vi "PPS User Interface.vi"() -> ()   [LabVIEW 2023, in "GUI.lvlib" / "Diagnostic.lvlib"]
uses:
  Diagnostic.lvlib
  HardwareAbstractionLayer_LVOOP/Database/SQL Public VI/Control/DB Options.ctl
  Control/PPS Configure UI.ctl
  HardwareAbstractionLayer_LVOOP/PowerSupply/Control/PPS Configure Data.ctl
  HardwareAbstractionLayer_LVOOP/PowerSupply/PowerSupply.lvclass
  HardwareAbstractionLayer_LVOOP/Database/Database.lvclass
panel:
  in  "Stop":bool caption="Blank"
  in  "Apply":bool caption="Blank"
  in  "PPS Driver":T1(ring)
  out "error out":errorcluster
  in  "error in":errorcluster
  in  "PPS Operation":T2(tab)
  in  "PowerSupply Instrument":T3(ring)
  out "Status":bool
  out "Self-Test Result Message":string
  in  "OCP Delays (S)":dbl=1.0 caption="Absolute Resolution (1E-6)" format="%.2p"
  in  "OVP Delays (S)":dbl=1.0 caption="Absolute Resolution (1E-6)" format="%.2p"
  in  "Current Limit OCP (A)":dbl=8.0 caption="Absolute Resolution (1E-6)" format="%.2p"
  in  "Voltage Limit  (V)":dbl=15.0 caption="Absolute Resolution (1E-6)" format="%.2p"
  in  "Current  Limit  (A)":dbl=6.0 caption="Absolute Resolution (1E-6)" format="%.2p"
  in  "Voltage Limit OVP (V)":dbl=15.0 caption="Absolute Resolution (1E-6)" format="%.2p"
  in  "Current Level (A)":dbl=8.0 caption="Absolute Resolution (1E-6)" format="%.2p"
  in  "Voltage Level (V)":dbl=12.0 format="%#.2g"
  in  "Output Priority Mode":u16(ring) items=["Voltage", "Current"]
  in  "Output":bool
  in  "OVP":bool
  in  "OCP":bool
  out "Current (A)":dbl format="%_4f"
  out "Voltage (V)":dbl format="%_4f"
  # "Programmbale Power Supply"
  # "Operation:"
  # "Self Test is Enabled by selecting this opeartion"
  # "PPS Close Operation will be executing \n        by selecting this opeartion"
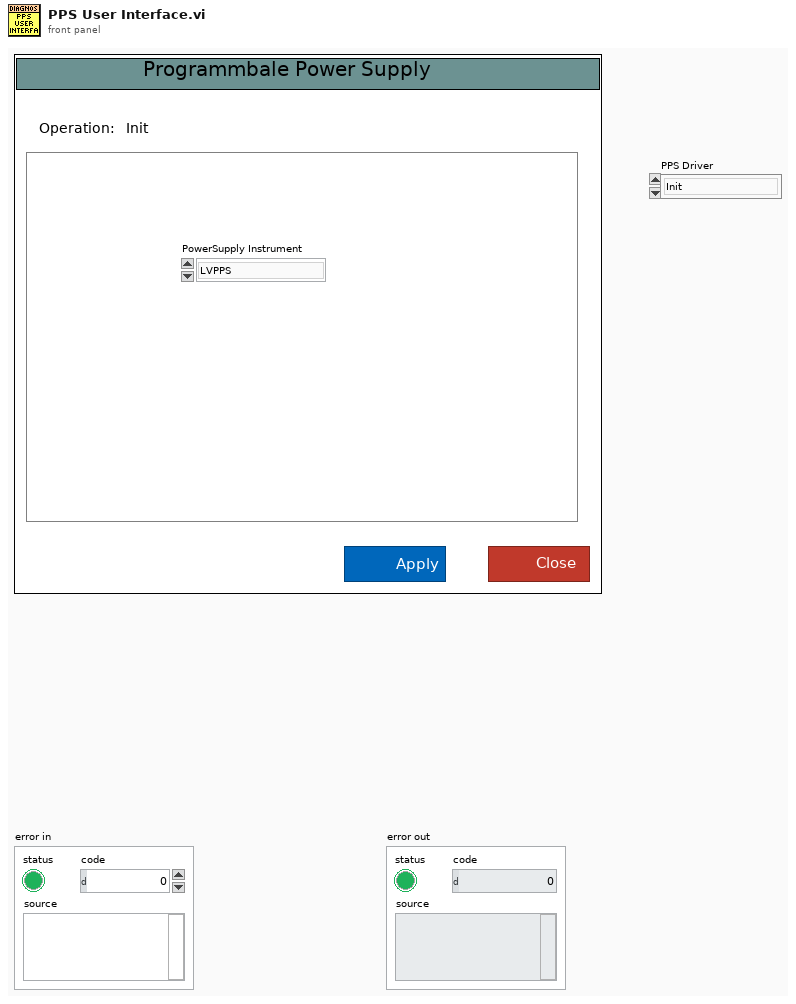
[diagram p1: front panel]
types:
  T1 = enum32{"Init", "Self Test", "Configure", "Measure", "Close"}
  T2 = enum32{"Init", "Self Test", "Configure", "Measure Current", "Measure Voltage", "Close"}
  T3 = enum16{"LVPPS", "HVPPS1", "HVPPS2", "HVPPS3", "HVPPS4", "HVPPS5", "HVPPS6"}
  T4 = typedef "HardwareAbstractionLayer_LVOOP.lvlib/Database.lvclass/DB Options.ctl" = enum16{"Init", "Select Data", "Insert Data", "Update Data", "Delete Data", "Execute Query", "Create Schema", "Create Table", "List Tables", "List Columns", "Close"}
  T5 = typedef "GUI.lvlib/Diagnostic.lvlib/PPS Configure UI.ctl" = cluster{"PPS Operation":enum32{"Init", "Self Test", "Configure", "Measure", "Close"}, "PowerSupply Instrument":enum16{"LVPPS", "HVPPS1", "HVPPS2", "HVPPS3", "HVPPS4", "HVPPS5", "HVPPS6"}, "Configure":T6}
  T6 = typedef "HardwareAbstractionLayer_LVOOP.lvlib/PowerSupply.lvclass/PPS Configure Data.ctl" = cluster{"Voltage Level (0.0 V)":dbl, "CURRent Limit (0.0 A)":dbl, "OVP LEVEL (0V)":dbl, "OCP LEVEL (0A)":dbl, "Enable OVP (T: Enable)":bool, "Enable OCP (T: Enable)":bool, "Enable Output ":bool, "Delays OCP":dbl, "Delays OVP":dbl, "Mode(0:Voltage)":u16, "CURRent Level (0.0 A)":dbl, "Voltage Limit (0.0 V)":dbl}
  T7 = typedef "GUI.lvlib/Diagnostic.lvlib/PPS Out Data UI.ctl" = cluster{"Self-Test Result Message":string, "Actual Voltage Level (V)":dbl, "Actual Current Limit (A)":dbl}
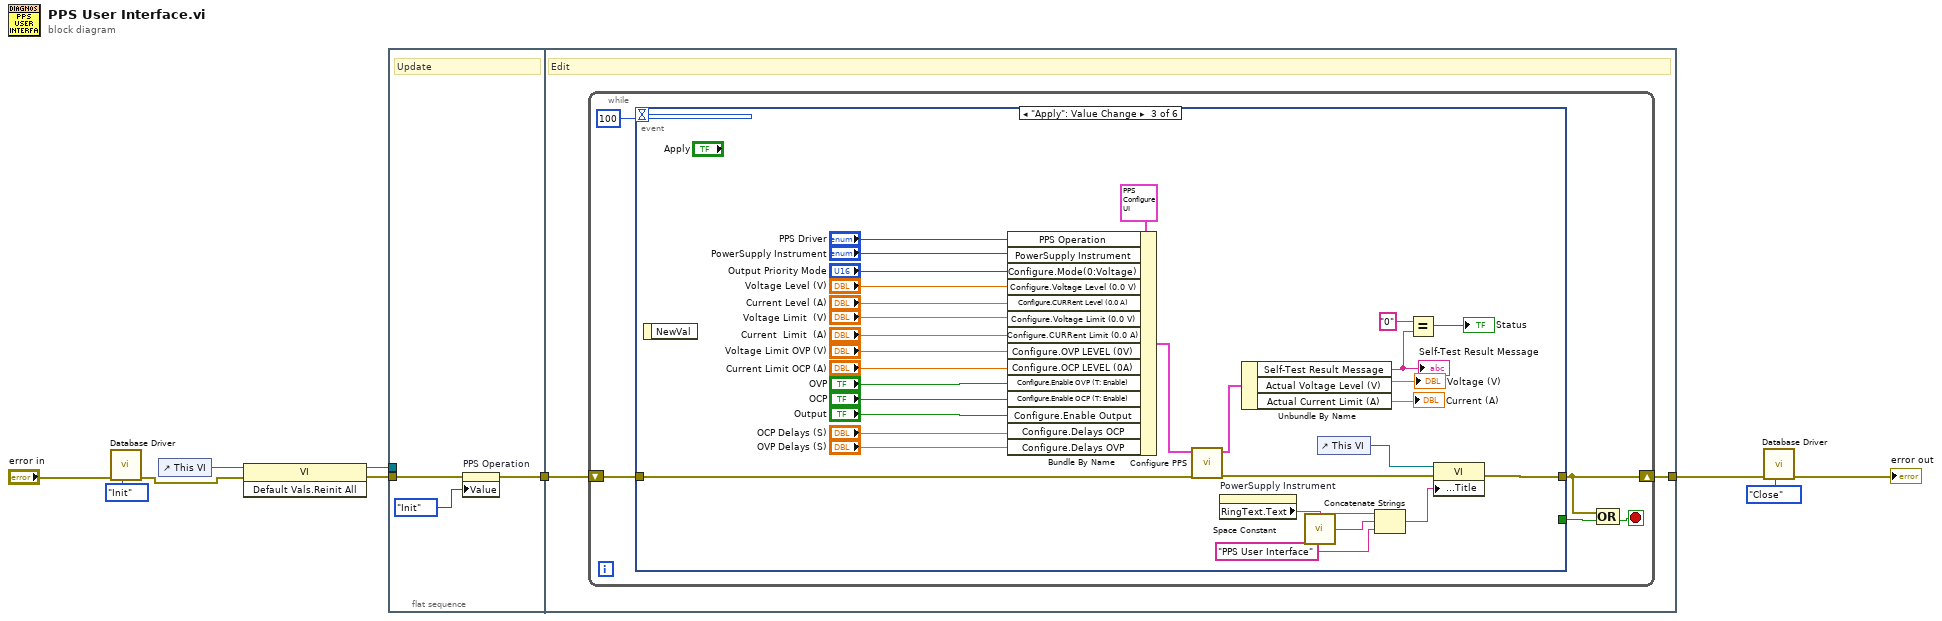
[diagram p0: block diagram]
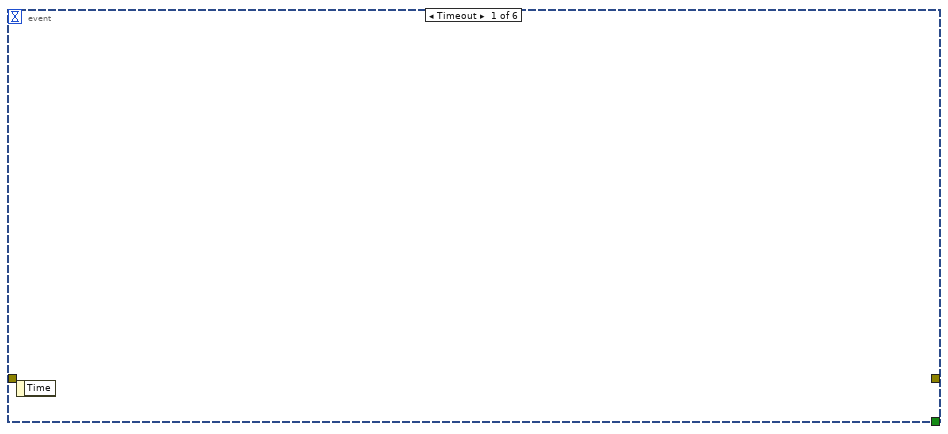
[diagram p2: hidden frame]
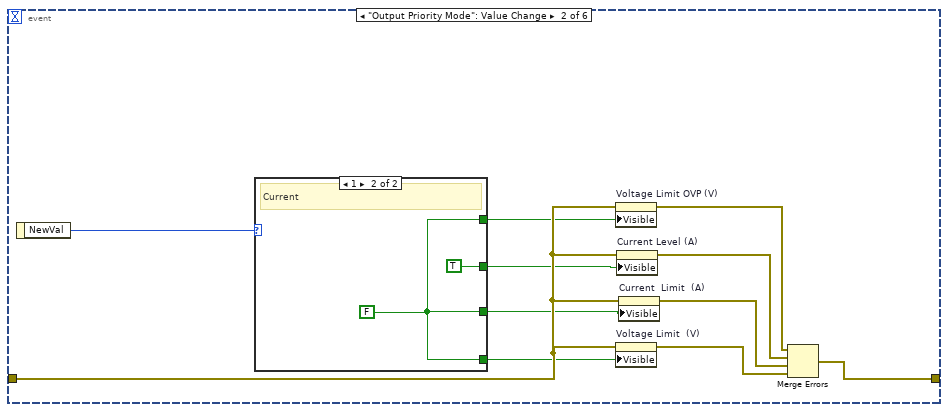
[diagram p3: hidden frame]
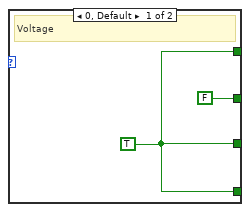
[diagram p4: hidden frame]
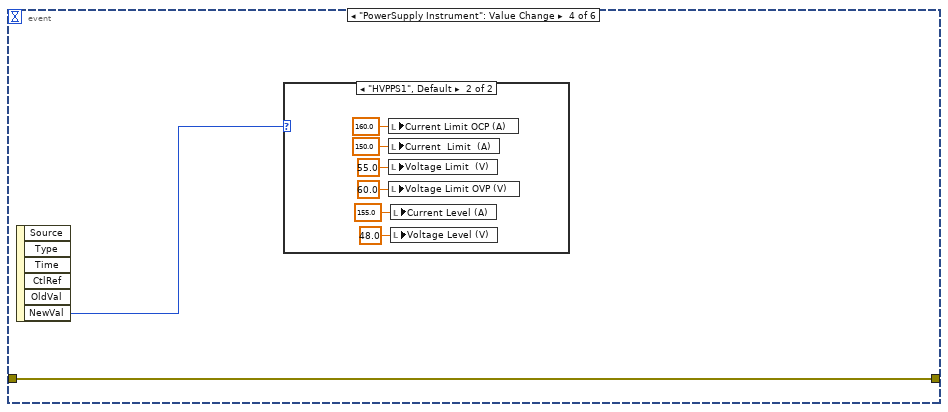
[diagram p5: hidden frame]
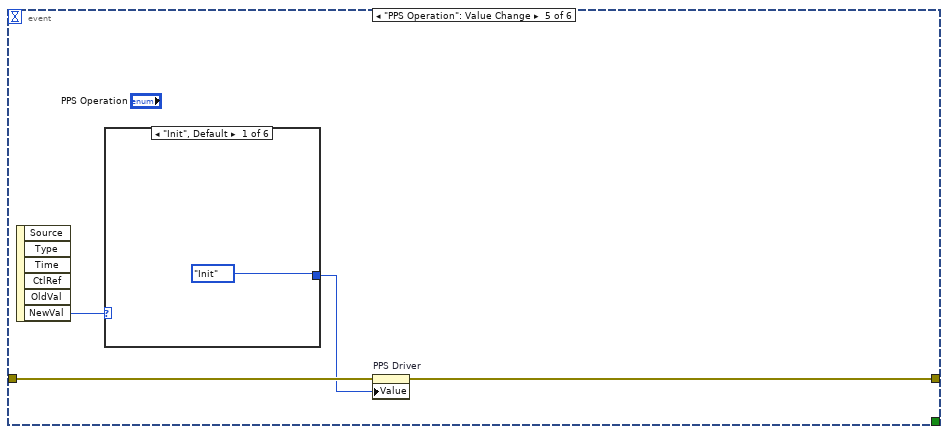
[diagram p7: hidden frame]
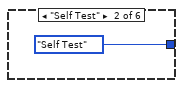
[diagram p8: hidden frame]
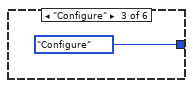
[diagram p9: hidden frame]
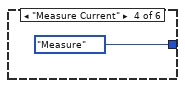
[diagram p10: hidden frame]
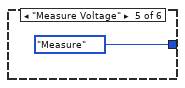
[diagram p11: hidden frame]
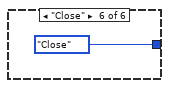
[diagram p12: hidden frame]
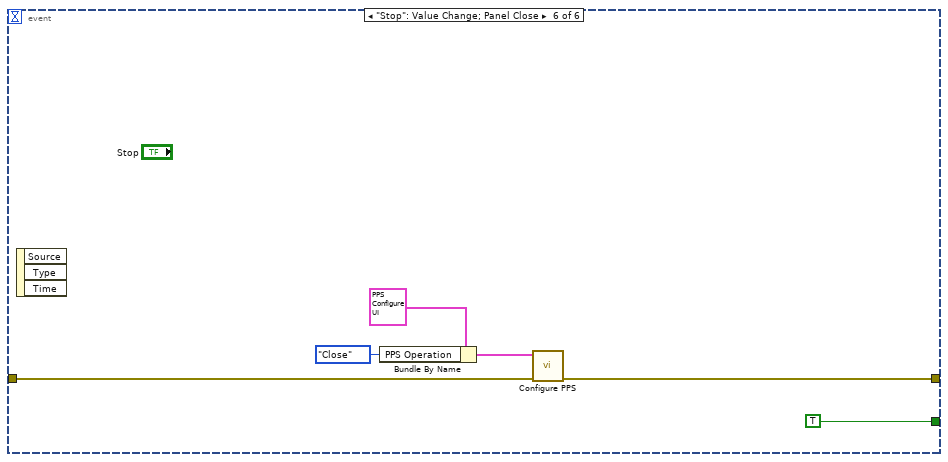
[diagram p13: hidden frame]
diagram:
  n1 = call "Database Driver.vi"("Options"=DB_Options."Init", "error in"="error in") -> ("error out"=w4:errorcluster)  [unwired: 6 in, 3 out]
  n2 = control-ref of="This VI"() -> (w10:refnum<vi>)
  n3 = invoke class="VI" method="Default Vals.Reinit All"(reference=w10, error in=w4) -> (reference out=w9:refnum<vi>, error out=w8:errorcluster)  [unwired: 1 in, 1 out]
  n4 = flat-sequence {
    tunnel: w9 -> [_]
    tunnel: w8 -> [w12]
    tunnel: [w11] -> w7
    tunnel: w7 -> [w15]
    tunnel: [w14] -> w6
    frame #0 {
      # "Update"
      n5 = property on="PPS Operation" class="TabCtl (strict)"(error in=w12, "Value"=T2."Init" ("PPS Operation")) -> (error out=w11:errorcluster)  [unwired: 1 in, 1 out]
    }
    frame #1 {
      # "Edit"
      n6 = while {
        shift-right: [w16] -> w14
        shift-left: w15 -> [w18]
        stop <- w17 stop-if-true
        n7 = event shown="[2] \"Apply\": Value Change" {
          selector: _ -> [_ _ _ _ _ _]
          dyn-events: _ -> [_ _ _ _ _ _]
          timeout: 100 -> [_ _ _ _ _ _]
          tunnel: [_ _ _ _ _ TRUE ("Stop")] -> w19
          tunnel: w18 -> [_ w30 w65 w66 w76 w88]
          tunnel: [_ w21 w40 w66 w75 w87] -> w16
          event Timeout {
            n8 = event-data() -> ()  [unwired: 1 in, 1 out]
          }
          event "Output Priority Mode": Value Change {
            n9 = event-data() -> ("NewVal"=w31:u16)  [unwired: 1 in]
            n10 = case shown="1" w31 {
              tunnel: [w32 w34] -> w29
              tunnel: [w32 w34] -> w28
              tunnel: [FALSE ("Visible") TRUE ("Visible")] -> w27
              tunnel: [w32 w34] -> w26
              frame 0, Default {
                w32 = TRUE ("Visible")
                # "Voltage"
              }
              frame 1 {
                w34 = FALSE ("Visible")
                # "Current"
              }
            }
            n11 = property on="Voltage Limit OVP (V)" class="DigNum (strict)"(error in=w30, "Visible"=w29) -> (error out=w25:errorcluster)  [unwired: 1 in, 1 out]
            n12 = property on="Voltage Limit  (V)" class="DigNum (strict)"(error in=w30, "Visible"=w28) -> (error out=w22:errorcluster)  [unwired: 1 in, 1 out]
            n13 = property on="Current Level (A)" class="DigNum (strict)"(error in=w30, "Visible"=w27) -> (error out=w24:errorcluster)  [unwired: 1 in, 1 out]
            n14 = property on="Current  Limit  (A)" class="DigNum (strict)"(error in=w30, "Visible"=w26) -> (error out=w23:errorcluster)  [unwired: 1 in, 1 out]
            n15 = Merge Errors(w25, w24, w23, w22) -> (w21:errorcluster)
          }
          event "Apply": Value Change {
            n16 = event-data() -> ()  [unwired: 1 in, 1 out]
            n17 = Bundle By Name(cluster=T5 {"PPS Operation"=enum."Close", "PowerSupply Instrument"=enum."LVPPS", "Configure"={"Voltage Level (0.0 V)"=0.0, "CURRent Limit (0.0 A)"=0.0, "OVP LEVEL (0V)"=0.0, "OCP LEVEL (0A)"=0.0, "Enable OVP (T: Enable)"=TRUE, "Enable OCP (T: Enable)"=TRUE, "Enable Output "=TRUE, "Delays OCP"=0.0, "Delays OVP"=0.0, "Mode(0:Voltage)"=0, "CURRent Level (0.0 A)"=0.0, "Voltage Limit (0.0 V)"=0.0}} ("PPS Config In"), "PPS Operation"="PPS Driver", "PowerSupply Instrument"="PowerSupply Instrument", "Configure.Mode(0:Voltage)"="Output Priority Mode", "Configure.Voltage Level (0.0 V)"="Voltage Level (V)", "Configure.CURRent Level (0.0 A)"="Current Level (A)", "Configure.Voltage Limit (0.0 V)"="Voltage Limit  (V)", "Configure.CURRent Limit (0.0 A)"="Current  Limit  (A)", "Configure.OVP LEVEL (0V)"="Voltage Limit OVP (V)", "Configure.OCP LEVEL (0A)"="Current Limit OCP (A)", "Configure.Enable OVP (T: Enable)"="OVP", "Configure.Enable OCP (T: Enable)"="OCP", "Configure.Enable Output"="Output", "Configure.Delays OCP"="OCP Delays (S)", "Configure.Delays OVP"="OVP Delays (S)") -> (w60:T5)
            n18 = call "Configure PPS.vi"("error in"=w65, "PPS Config In"=w60) -> ("error out"=w41:errorcluster, "PPS Out"=w64:T7)  [unwired: 8 in]
            n19 = property on="PowerSupply Instrument" class="Enum (strict)"() -> ("RingText.Text"=w39:string)  [unwired: 2 in, 2 out]
            n20 = Unbundle By Name(w64) -> ("Self-Test Result Message"=w46:string, "Actual Voltage Level (V)"=→"Voltage (V)":dbl, "Actual Current Limit (A)"=→"Current (A)":dbl)
            "Self-Test Result Message" <- w46
            n21 = call <vilib>:"Space Constant.vi"() -> ("String"=w36:string)
            n22 = control-ref of="This VI"() -> (w42:refnum<vi>)
            n23 = Concatenate Strings(w39, w36, "PPS User Interface") -> (w38:string)
            n24 = Equal?(x="0", y=w46) -> (x = y?=→"Status":bool)
            n25 = property class="VI"(reference=w42, error in=w41, "Front Panel.Title"=w38) -> (error out=w40:errorcluster)  [unwired: 1 out]
          }
          event "PowerSupply Instrument": Value Change {
            n26 = event-data() -> ("NewVal"=w67:T3)  [unwired: 1 in, 5 out]
            n27 = case shown="\"HVPPS1\", Default" w67 {
              frame "LVPPS" {
              }
              frame "HVPPS1", Default {
                n28 = local write "Current Limit OCP (A)"(160.0 ("Current Limit OCP (A)")) -> ()
                n29 = local write "Current  Limit  (A)"(150.0 ("Current  Limit  (A)")) -> ()
                n30 = local write "Voltage Limit  (V)"(55.0 ("Voltage Limit  (V)")) -> ()
                n31 = local write "Voltage Limit OVP (V)"(60.0 ("Voltage Limit OVP (V)")) -> ()
                n32 = local write "Current Level (A)"(155.0 ("Current Level (A)")) -> ()
                n33 = local write "Voltage Level (V)"(48.0 ("Voltage Level (V)")) -> ()
              }
            }
          }
          event "PPS Operation": Value Change {
            n34 = event-data() -> ("NewVal"=w77:T2)  [unwired: 1 in, 5 out]
            n35 = case shown="\"Init\", Default" w77 {
              tunnel: [T1."Init" ("PPS Driver") T1."Self Test" ("PPS Driver") T1."Configure" ("PPS Driver") T1."Measure" ("PPS Driver") T1."Measure" ("PPS Driver") T1."Close" ("PPS Driver")] -> w74
              frame "Init", Default {
              }
              frame "Self Test" {
              }
              frame "Configure" {
              }
              frame "Measure Current" {
              }
              frame "Measure Voltage" {
              }
              frame "Close" {
              }
            }
            n36 = property on="PPS Driver" class="Enum (strict)"(error in=w76, "Value"=w74) -> (error out=w75:errorcluster)  [unwired: 1 in, 1 out]
          }
          event "Stop": Value Change; Panel Close {
            n37 = event-data() -> ()  [unwired: 1 in, 3 out]
            n38 = Bundle By Name(cluster=T5 {"PPS Operation"=enum."Close", "PowerSupply Instrument"=enum."LVPPS", "Configure"={"Voltage Level (0.0 V)"=0.0, "CURRent Limit (0.0 A)"=0.0, "OVP LEVEL (0V)"=0.0, "OCP LEVEL (0A)"=0.0, "Enable OVP (T: Enable)"=TRUE, "Enable OCP (T: Enable)"=TRUE, "Enable Output "=TRUE, "Delays OCP"=0.0, "Delays OVP"=0.0, "Mode(0:Voltage)"=0, "CURRent Level (0.0 A)"=0.0, "Voltage Limit (0.0 V)"=0.0}} ("PPS Config In"), "PPS Operation"=T1."Close") -> (w85:T5)
            n39 = call "Configure PPS.vi"("error in"=w88, "PPS Config In"=w85) -> ("error out"=w87:errorcluster)  [unwired: 8 in, 1 out]
          }
        }
        n40 = Compound Arithmetic op=OR(w16, w19) -> (w17:bool)
      }
    }
  }
  n41 = call "Database Driver.vi"("Options"=DB_Options."Close", "error in"=w6) -> ("error out"=→"error out":errorcluster)  [unwired: 6 in, 3 out]
